vi "Detect LR.vi"(9 "Side Gyro Data":T1={"Time"=0.0, "Gyro Array Data"=[], "Gyro Negation"=[], "Gyro Data"={"Gyro X"=0.0, "Gyro Y"=0.0, "Gyro Z"=0.0}, "Gyro Latency"=0.0, "Normalization Time"=640.0, "Sampling Rate"=0.0}, 10 "Side Event Data":T3={"Event Data"={"LR"={"Phase"="LR", "On"=FALSE, "Last On Time"=0.0, "Duration"=0.0, "Crossing Time"=0.0, "Time since LR"=0.0, "Time Since TSw"=0.0, "Min gyro Z"=0.0, "Time since LR?"=FALSE, "Time since TSw?"=FALSE, "Min gyro Z?"=FALSE, "Crossing?"=FALSE}, "MSt"={"Phase"="MSt", "On"=FALSE, "Last On Time"=0.0, "Duration"=0.0}, "TSt"={"Phase"="TSt", "On"=FALSE, "Last On Time"=0.0, "Duration"=0.0}, "PSw"={"Phase"="PSw", "On"=FALSE, "Last On Time"=0.0, "Duration"=0.0}, "ISw"={"Phase"="ISw", "On"=FALSE, "Last On Time"=0.0, "Duration"=0.0, "Peak Time"=0.0, "Time since LR"=0.0, "Time since ISw"=0.0, "Time since LR?"=FALSE, "Time since ISw?"=FALSE, "Peak?"=FALSE}, "MSw"={"Phase"="MSw", "On"=FALSE, "Last On Time"=0.0, "Duration"=0.0, "Crossing time"=0.0, "Time since LR"=0.0, "Time since MSw"=0.0, "Time since ISw"=0.0, "Time since LR?"=FALSE, "Time since MSw?"=FALSE, "Time since ISw?"=FALSE, "Crossing?"=FALSE}, "TSw"={"Phase"="TSw", "On"=FALSE, "Last On Time"=0.0, "Duration"=0.0, "Peak time"=0.0, "Time since LR"=0.0, "Time since TSw"=0.0, "Time since LR?"=FALSE, "Time since TSw?"=FALSE, "Peak?"=FALSE}}, "Mean Cycle Duration"=0.0, "Event Detected?"=FALSE, "Last Event Detected"=0, "Num Cycles"=0.0, "GPD Log"=refnum, "Last Event Time"=0.0}, 11 "GPD Parameters":T4={"% Cycle Delay"=0.0, "Min % Cycle LR to ISw "=0.0, "Min % Cycle LR to MSw"=0.0, "Min % Cycle LR to TSw"=0.0, "Max % Cycle ISw to MSw"=0.0, "Min % Cycle TSw to LR"=0.0, "Max % Cycle TSw to LR"=0.0, "LR Min Gyro Z Threshold"=0.0, "LR Min Gyro Z Width"=0.0, "ISw Peak Threshold"=0.0, "ISw Peak Width"=0.0, "TSw Valley Threshold"=0.0, "TSw Valley Width (ms)"=7.0, "Max Cycle Time (s)"=0.0, "Mean Computation Window"=0.0, "CP subject?"=FALSE}) -> (1 "Side Gyro Data":T1={"Time"=0.0, "Gyro Array Data"=[], "Gyro Negation"=[], "Gyro Data"={"Gyro X"=0.0, "Gyro Y"=0.0, "Gyro Z"=0.0}, "Gyro Latency"=0.0, "Normalization Time"=640.0, "Sampling Rate"=0.0}, 2 "Side Event Data":T3={"Event Data"={"LR"={"Phase"="LR", "On"=FALSE, "Last On Time"=0.0, "Duration"=0.0, "Crossing Time"=0.0, "Time since LR"=0.0, "Time Since TSw"=0.0, "Min gyro Z"=0.0, "Time since LR?"=FALSE, "Time since TSw?"=FALSE, "Min gyro Z?"=FALSE, "Crossing?"=FALSE}, "MSt"={"Phase"="MSt", "On"=FALSE, "Last On Time"=0.0, "Duration"=0.0}, "TSt"={"Phase"="TSt", "On"=FALSE, "Last On Time"=0.0, "Duration"=0.0}, "PSw"={"Phase"="PSw", "On"=FALSE, "Last On Time"=0.0, "Duration"=0.0}, "ISw"={"Phase"="ISw", "On"=FALSE, "Last On Time"=0.0, "Duration"=0.0, "Peak Time"=0.0, "Time since LR"=0.0, "Time since ISw"=0.0, "Time since LR?"=FALSE, "Time since ISw?"=FALSE, "Peak?"=FALSE}, "MSw"={"Phase"="MSw", "On"=FALSE, "Last On Time"=0.0, "Duration"=0.0, "Crossing time"=0.0, "Time since LR"=0.0, "Time since MSw"=0.0, "Time since ISw"=0.0, "Time since LR?"=FALSE, "Time since MSw?"=FALSE, "Time since ISw?"=FALSE, "Crossing?"=FALSE}, "TSw"={"Phase"="TSw", "On"=FALSE, "Last On Time"=0.0, "Duration"=0.0, "Peak time"=0.0, "Time since LR"=0.0, "Time since TSw"=0.0, "Time since LR?"=FALSE, "Time since TSw?"=FALSE, "Peak?"=FALSE}}, "Mean Cycle Duration"=0.0, "Event Detected?"=FALSE, "Last Event Detected"=0, "Num Cycles"=0.0, "GPD Log"=refnum, "Last Event Time"=0.0}, 3 "GPD Parameters":T4={"% Cycle Delay"=0.0, "Min % Cycle LR to ISw "=0.0, "Min % Cycle LR to MSw"=0.0, "Min % Cycle LR to TSw"=0.0, "Max % Cycle ISw to MSw"=0.0, "Min % Cycle TSw to LR"=0.0, "Max % Cycle TSw to LR"=0.0, "LR Min Gyro Z Threshold"=0.0, "LR Min Gyro Z Width"=0.0, "ISw Peak Threshold"=0.0, "ISw Peak Width"=0.0, "TSw Valley Threshold"=0.0, "TSw Valley Width (ms)"=7.0, "Max Cycle Time (s)"=0.0, "Mean Computation Window"=0.0, "CP subject?"=FALSE}, 4 "LR Detected?":bool)   [LabVIEW 2019]
uses:
  Controls/Gyro Side Data.ctl
  Controls/Gyro Negation.ctl
  Controls/GPD Side Parameters.ctl
  Controls/Side Event Data.ctl
  <vilib>/ptbypt/NI_PtbyPt.lvlib
panel:
  out "LR at about 7 sec":bool
  out "output cluster":T5
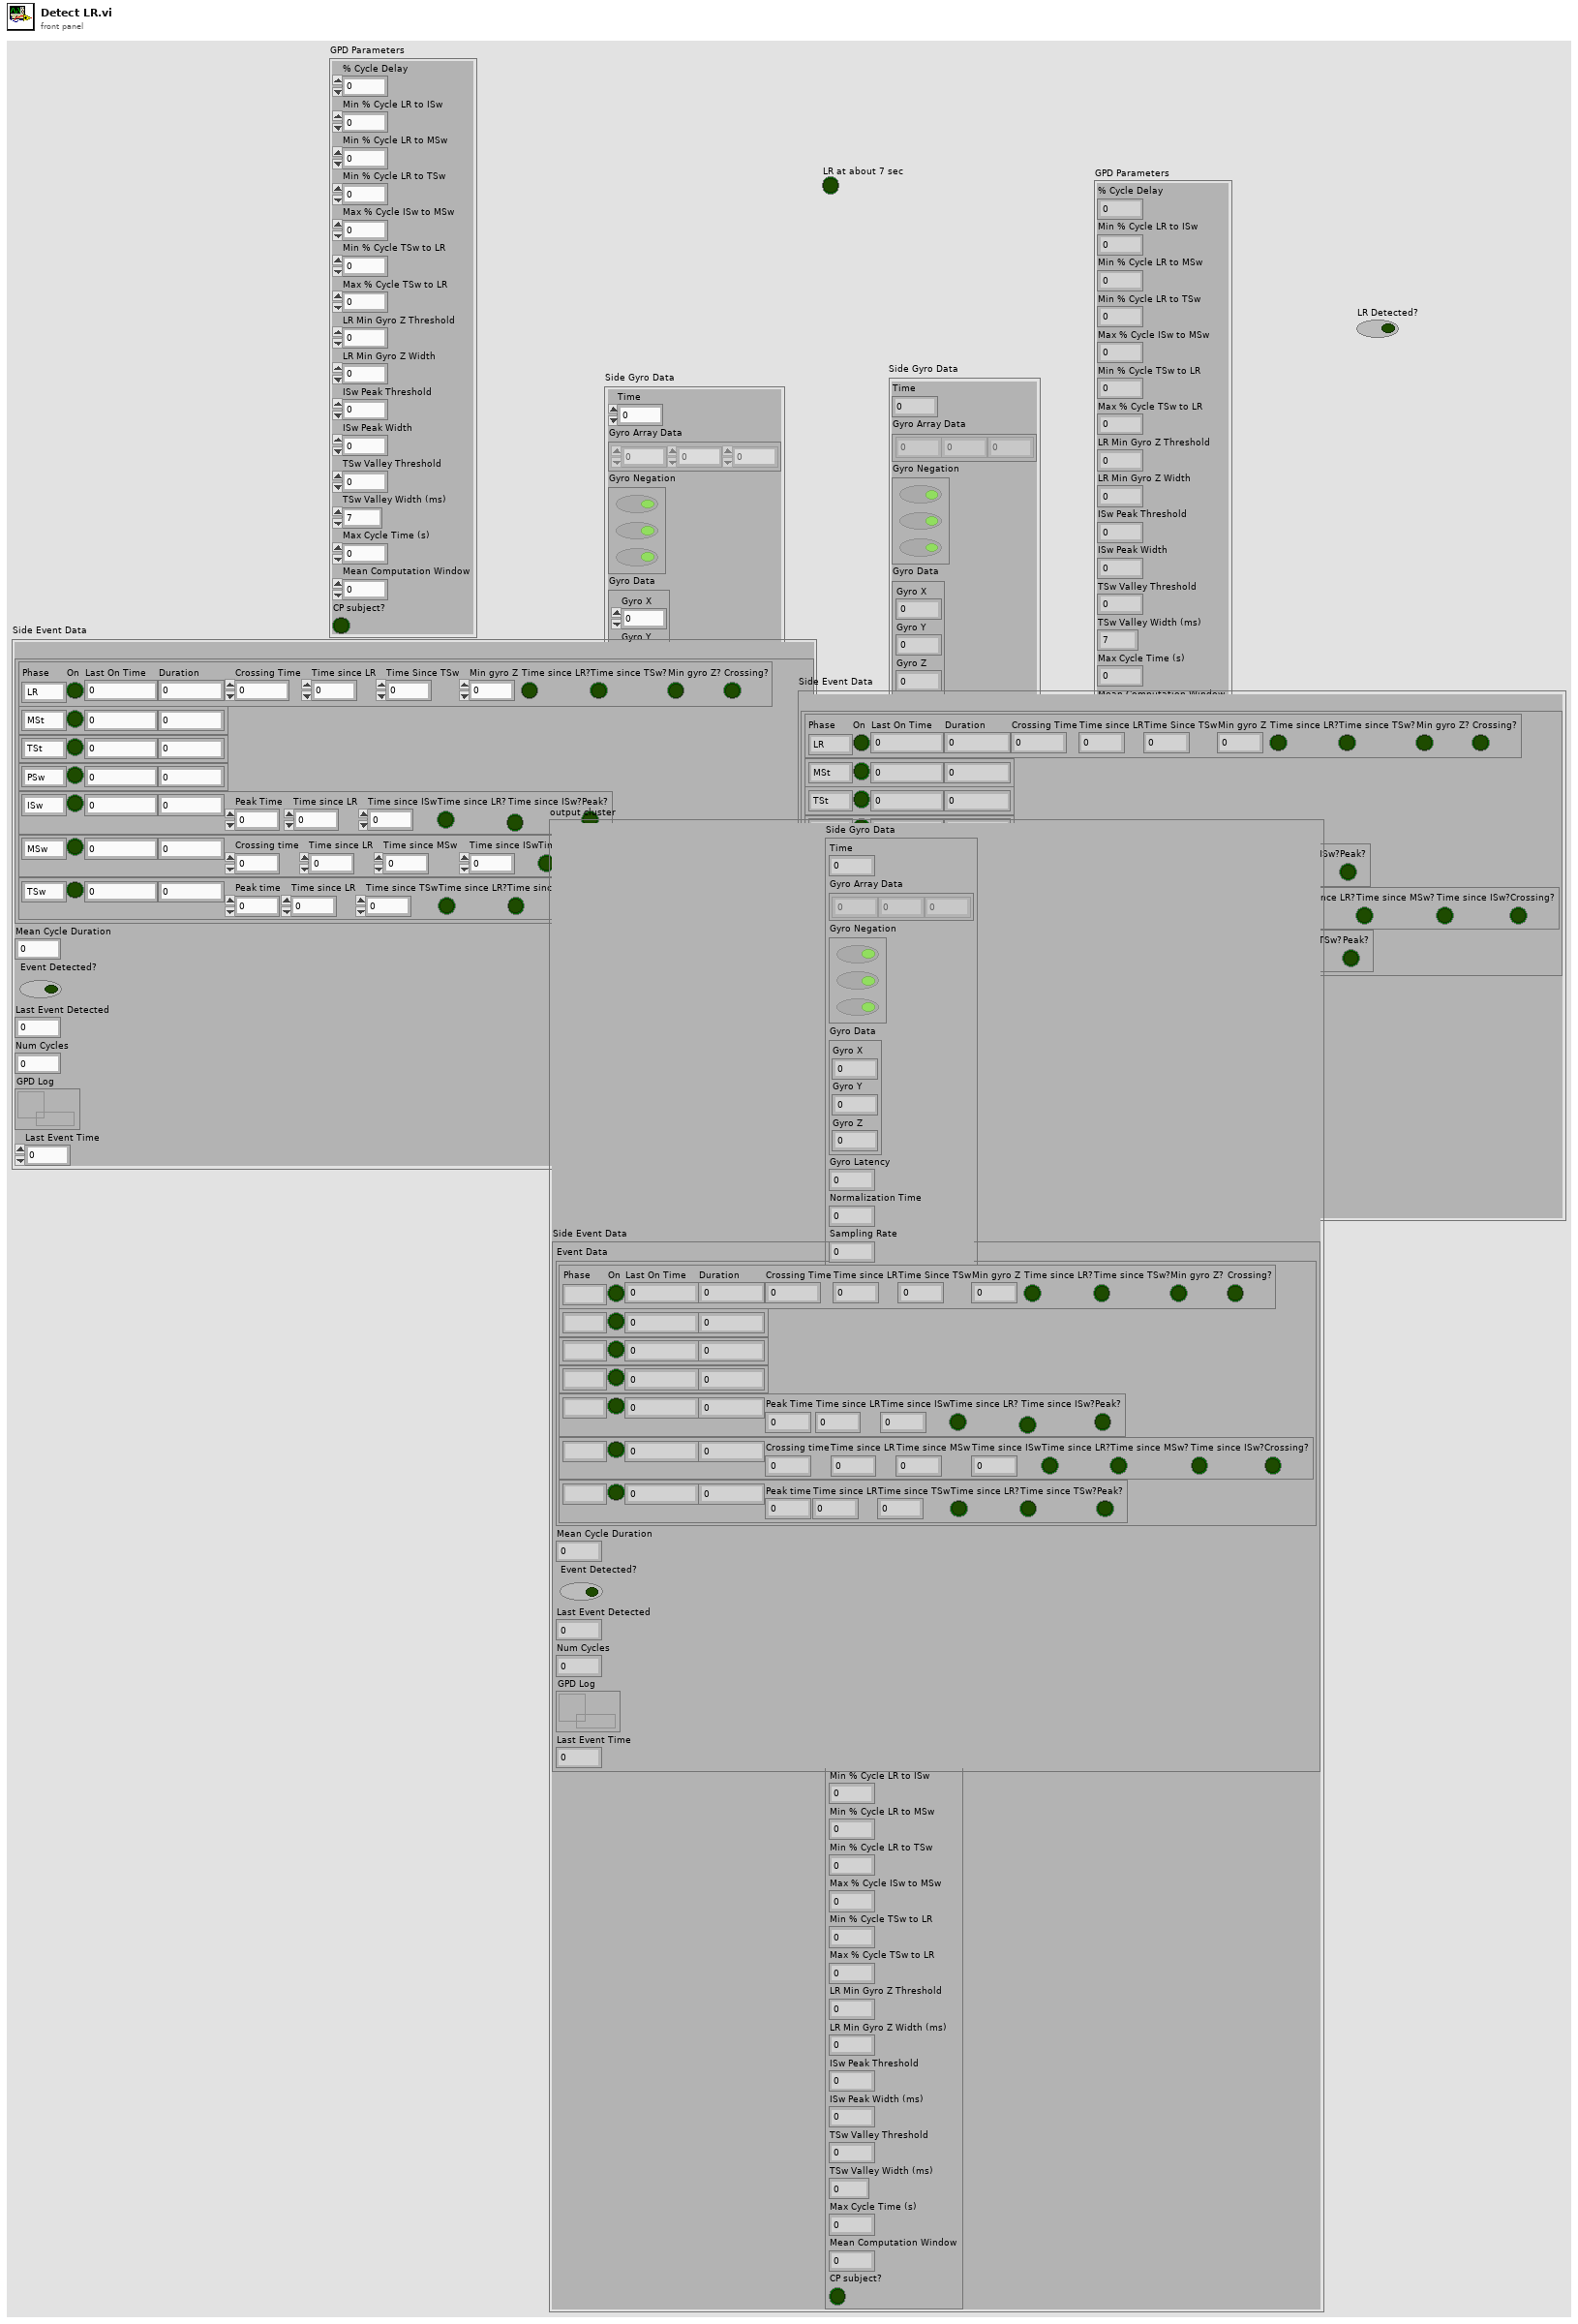
[diagram p1: front panel]
types:
  T1 = typedef "Gyro Side Data.ctl" = cluster{"Time":dbl, "Gyro Array Data":dbl[], "Gyro Negation":T2, "Gyro Data":cluster{"Gyro X":dbl, "Gyro Y":dbl, "Gyro Z":dbl}, "Gyro Latency":dbl, "Normalization Time":dbl, "Sampling Rate":dbl}
  T2 = typedef "Gyro Negation.ctl" = bool[]
  T3 = typedef "Side Event Data.ctl" = cluster{"Event Data":cluster{"LR":cluster{"Phase":string, "On":bool, "Last On Time":dbl, "Duration":dbl, "Crossing Time":dbl, "Time since LR":dbl, "Time Since TSw":dbl, "Min gyro Z":dbl, "Time since LR?":bool, "Time since TSw?":bool, "Min gyro Z?":bool, "Crossing?":bool}, "MSt":cluster{"Phase":string, "On":bool, "Last On Time":dbl, "Duration":dbl}, "TSt":cluster{"Phase":string, "On":bool, "Last On Time":dbl, "Duration":dbl}, "PSw":cluster{"Phase":string, "On":bool, "Last On Time":dbl, "Duration":dbl}, "ISw":cluster{"Phase":string, "On":bool, "Last On Time":dbl, "Duration":dbl, "Peak Time":dbl, "Time since LR":dbl, "Time since ISw":dbl, "Time since LR?":bool, "Time since ISw?":bool, "Peak?":bool}, "MSw":cluster{"Phase":string, "On":bool, "Last On Time":dbl, "Duration":dbl, "Crossing time":dbl, "Time since LR":dbl, "Time since MSw":dbl, "Time since ISw":dbl, "Time since LR?":bool, "Time since MSw?":bool, "Time since ISw?":bool, "Crossing?":bool}, "TSw":cluster{"Phase":string, "On":bool, "Last On Time":dbl, "Duration":dbl, "Peak time":dbl, "Time since LR":dbl, "Time since TSw":dbl, "Time since LR?":bool, "Time since TSw?":bool, "Peak?":bool}}, "Mean Cycle Duration":dbl, "Event Detected?":bool, "Last Event Detected":i32, "Num Cycles":dbl, "GPD Log":refnum<queue>, "Last Event Time":dbl}
  T4 = typedef "GPD Side Parameters.ctl" = cluster{"% Cycle Delay":dbl, "Min % Cycle LR to ISw ":dbl, "Min % Cycle LR to MSw":dbl, "Min % Cycle LR to TSw":dbl, "Max % Cycle ISw to MSw":dbl, "Min % Cycle TSw to LR":dbl, "Max % Cycle TSw to LR":dbl, "LR Min Gyro Z Threshold":dbl, "LR Min Gyro Z Width":dbl, "ISw Peak Threshold":dbl, "ISw Peak Width":dbl, "TSw Valley Threshold":dbl, "TSw Valley Width (ms)":dbl, "Max Cycle Time (s)":dbl, "Mean Computation Window":dbl, "CP subject?":bool}
  T5 = cluster{"Side Gyro Data":T1, "Side Event Data":T3, "GPD Parameters":T4}
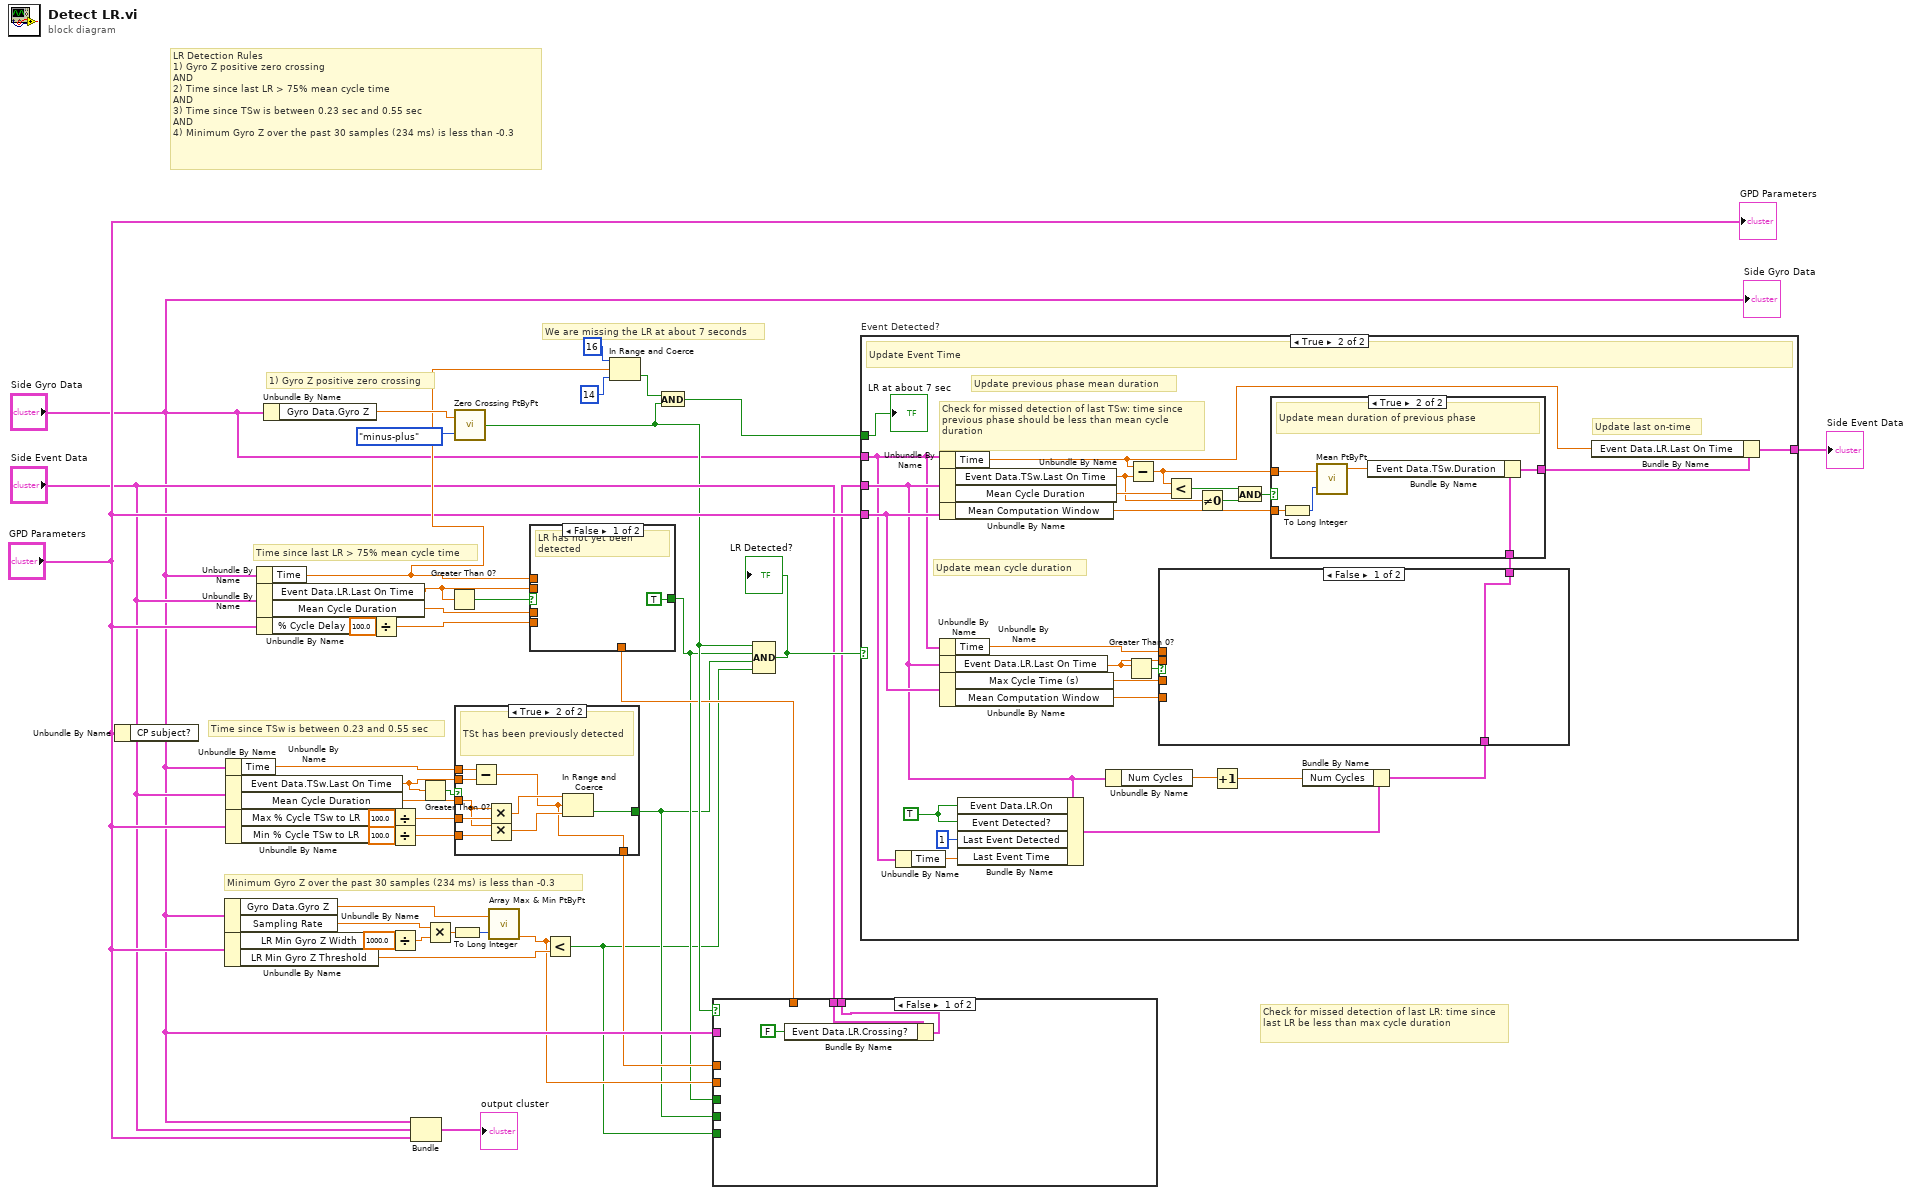
[diagram p0: block diagram]
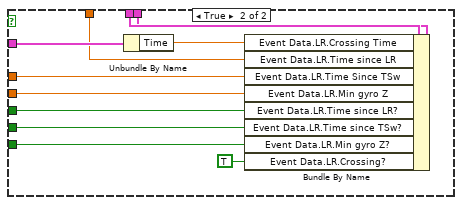
[diagram p2: hidden frame]
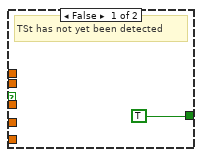
[diagram p3: hidden frame]
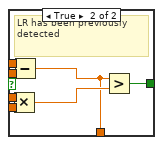
[diagram p4: hidden frame]
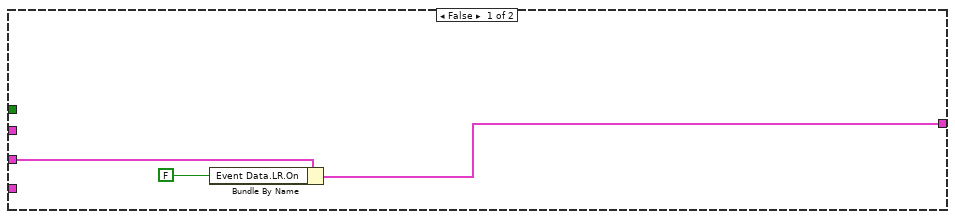
[diagram p5: hidden frame]
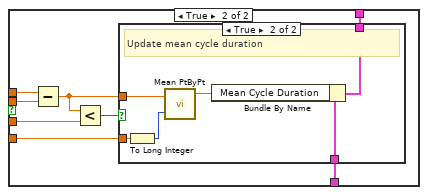
[diagram p6: hidden frame]
diagram:
  # "Check for missed detection of last LR: time since last LR be less than max cycle duration"
  # "Minimum Gyro Z over the past 30 samples (234 ms) is less than -0.3"
  # "Time since TSw is between 0.23 and 0.55 sec"
  # "Time since last LR > 75% mean cycle time"
  # "We are missing the LR at about 7 seconds"
  # "1) Gyro Z positive zero crossing"
  # "LR Detection Rules\n1) Gyro Z positive zero crossing\nAND\n2) Time since last LR > 75% mean cycle time\nAND\n3) Time since TSw is between 0.23 sec and 0.55 sec\nAND\n4) Minimum Gyro Z over the past 30 samples (234 ms) is less than -0.3"
  n1 = Unbundle By Name("GPD Parameters") -> ()  [unwired: 1 out]
  n2 = Unbundle By Name("Side Gyro Data") -> ("Gyro Data.Gyro Z"=w20:dbl, "Sampling Rate"=w16:dbl)
  n3 = Unbundle By Name("GPD Parameters") -> ("LR Min Gyro Z Width"=w18:dbl, "LR Min Gyro Z Threshold"=w13:dbl)
  n4 = Unbundle By Name("Side Gyro Data") -> ("Time"=w28:dbl)
  n5 = Unbundle By Name("Side Event Data") -> ("Event Data.TSw.Last On Time"=w11:dbl, "Mean Cycle Duration"=w22:dbl)
  n6 = Unbundle By Name("GPD Parameters") -> ("Max % Cycle TSw to LR"=w25:dbl, "Min % Cycle TSw to LR"=w24:dbl)
  n7 = Unbundle By Name("Side Gyro Data") -> ("Time"=w31:dbl)
  n8 = Unbundle By Name("Side Event Data") -> ("Event Data.LR.Last On Time"=w37:dbl, "Mean Cycle Duration"=w34:dbl)
  n9 = Unbundle By Name("GPD Parameters") -> ("% Cycle Delay"=w33:dbl)
  n10 = Unbundle By Name("Side Gyro Data") -> ("Gyro Data.Gyro Z"=w43:dbl)
  n11 = Divide(x=w33, y=100.0) -> (x/y=w35:dbl)
  n12 = Divide(x=w25, y=100.0) -> (x/y=w23:dbl)
  n13 = Divide(x=w24, y=100.0) -> (x/y=w21:dbl)
  n14 = Divide(x=w18, y=1000.0) -> (x/y=w17:dbl)
  n15 = Bundle("Side Gyro Data"="Side Gyro Data", "Side Event Data"="Side Event Data", "GPD Parameters"="GPD Parameters") -> (→"output cluster":T5)  [unwired: 1 in]
  n16 = Greater Than 0?(x=w11) -> (x > 0?=w12:bool)
  n17 = Multiply(x=w16, y=w17) -> (x*y=w15:dbl)
  n18 = Greater Than 0?(x=w37) -> (x > 0?=w36:bool)
  n19 = To Long Integer(number=w15) -> (32bit integer=w14:i32)
  n20 = call <vilib>:"Zero Crossing PtByPt.vi"("direction"=enum16{"either", "minus-plus", "plus-minus"}."minus-plus", "input data point"=w43) -> ("crossing"=w8:bool)  [unwired: 1 in]
  n21 = case shown="True" w12 {
    tunnel: w28 -> [_ w55]
    tunnel: w11 -> [_ w54]
    tunnel: w23 -> [_ w53]
    tunnel: w22 -> [_ w52]
    tunnel: w21 -> [_ w51]
    tunnel: [TRUE w48] -> w2
    tunnel: [_ w47] -> w5
    frame False {
      # "TSt has not yet been detected"
    }
    frame True {
      # "TSt has been previously detected"
      n22 = Subtract(x=w55, y=w54) -> (x-y=w47:dbl)
      n23 = Multiply(x=w52, y=w53) -> (x*y=w50:dbl)
      n24 = Multiply(x=w52, y=w51) -> (x*y=w49:dbl)
      n25 = In Range and Coerce(upper limit=w50, x=w47, lower limit=w49) -> (In Range?=w48:bool)  [unwired: 1 out]
    }
  }
  n26 = call <vilib>:"Array Max & Min PtByPt.vi"("input data point"=w20, "sample length"=w14) -> ("min value"=w4:dbl)  [unwired: 1 in, 4 out]
  n27 = case shown="False" w36 {
    tunnel: w34 -> [_ w63]
    tunnel: w35 -> [_ w62]
    tunnel: w31 -> [_ w61]
    tunnel: w37 -> [_ w60]
    tunnel: [TRUE w59] -> w3
    tunnel: [_ w57] -> w6
    frame False {
      # "LR has not yet been detected"
    }
    frame True {
      # "LR has been previously detected"
      n28 = Multiply(x=w63, y=w62) -> (x*y=w58:dbl)
      n29 = Subtract(x=w61, y=w60) -> (x-y=w57:dbl)
      n30 = Greater?(x=w57, y=w58) -> (0:w59:bool)
    }
  }
  n31 = Less?(x=w4, y=w13) -> (x < y?=w1:bool)
  n32 = In Range and Coerce(upper limit=16, x=w31, lower limit=14) -> (In Range?=w39:bool)  [unwired: 1 out]
  n33 = And(x=w39, y=w8) -> (x .and. y?=w38:bool)
  n34 = case shown="False" w8 {
    tunnel: "Side Event Data" -> [w65 w77]
    tunnel: [w64 w76] -> w9
    tunnel: "Side Gyro Data" -> [_ w75]
    tunnel: w6 -> [_ w73]
    tunnel: w5 -> [_ w72]
    tunnel: w4 -> [_ w71]
    tunnel: w3 -> [_ w70]
    tunnel: w2 -> [_ w69]
    tunnel: w1 -> [_ w68]
    frame False {
      n35 = Bundle By Name(cluster=w65, "Event Data.LR.Crossing?"=FALSE) -> (w64:T3)
    }
    frame True {
      n36 = Unbundle By Name(w75) -> ("Time"=w74:dbl)
      n37 = Bundle By Name(cluster=w77, "Event Data.LR.Crossing Time"=w74, "Event Data.LR.Time since LR"=w73, "Event Data.LR.Time Since TSw"=w72, "Event Data.LR.Min gyro Z"=w71, "Event Data.LR.Time since LR?"=w70, "Event Data.LR.Time since TSw?"=w69, "Event Data.LR.Min gyro Z?"=w68, "Event Data.LR.Crossing?"=TRUE) -> (w76:T3)
    }
  }
  n38 = Compound Arithmetic op=AND(w8, w3, w2, w1) -> (w30:bool)
  "LR Detected?" <- w30
  n39 = case "Event Detected?" shown="True" w30 {
    tunnel: w9 -> [w80 w92]
    tunnel: [w79 w96] -> w45
    tunnel: "Side Gyro Data" -> [_ w84]
    tunnel: "GPD Parameters" -> [_ w100]
    tunnel: w38 -> [_ w83]
    frame False {
      n40 = Bundle By Name(cluster=w80, "Event Data.LR.On"=FALSE) -> (w79:T3)
    }
    frame True {
      w106 = TRUE
      # "Update last on-time"
      # "Check for missed detection of last TSw: time since previous phase should be less than mean cycle duration"
      # "Update mean cycle duration"
      # "Update previous phase mean duration"
      # "Update Event Time"
      n41 = Unbundle By Name(w84) -> ("Time"=w85:dbl)
      n42 = Unbundle By Name(w84) -> ("Time"=w104:dbl)
      n43 = Unbundle By Name(w92) -> ("Event Data.TSw.Last On Time"=w86:dbl, "Mean Cycle Duration"=w90:dbl)
      n44 = Unbundle By Name(w100) -> ("Mean Computation Window"=w94:dbl)
      n45 = Unbundle By Name(w84) -> ("Time"=w101:dbl)
      n46 = Unbundle By Name(w92) -> ("Event Data.LR.Last On Time"=w81:dbl)
      n47 = Unbundle By Name(w100) -> ("Max Cycle Time (s)"=w99:dbl, "Mean Computation Window"=w93:dbl)
      n48 = Bundle By Name(cluster=w92, "Event Data.LR.On"=w106, "Event Detected?"=w106, "Last Event Detected"=1, "Last Event Time"=w85) -> (w103:T3)
      n49 = Unbundle By Name(w92) -> ("Num Cycles"=w91:dbl)
      n50 = Greater Than 0?(x=w81) -> (x > 0?=w82:bool)
      n51 = Subtract(x=w104, y=w86) -> (x-y=w107:dbl)
      n52 = Less?(x=w107, y=w90) -> (x < y?=w88:bool)
      n53 = Not Equal To 0?(x=w86) -> (x != 0?=w89:bool)
      n54 = Increment(x=w91) -> (x+1=w102:dbl)
      n55 = And(x=w88, y=w89) -> (x .and. y?=w87:bool)
      n56 = Bundle By Name(cluster=w103, "Num Cycles"=w102) -> (w98:T3)
      n57 = case shown="False" w82 {
        tunnel: w101 -> [_ w116]
        tunnel: w81 -> [_ w115]
        tunnel: w99 -> [_ w114]
        tunnel: w98 -> [w108 w111]
        tunnel: [w108 w110] -> w97
        tunnel: w93 -> [_ w109]
        frame False {
        }
        frame True {
          n58 = Subtract(x=w116, y=w115) -> (x-y=w112:dbl)
          n59 = Less?(x=w112, y=w114) -> (x < y?=w113:bool)
          n60 = case shown="True" w113 {
            tunnel: w112 -> [_ w123]
            tunnel: w111 -> [w117 w122]
            tunnel: [w117 w120] -> w110
            tunnel: w109 -> [_ w119]
            frame False {
            }
            frame True {
              # "Update mean cycle duration"
              n61 = To Long Integer(number=w119) -> (32bit integer=w118:i32)
              n62 = call <vilib>:"Mean PtByPt.vi"("x"=w123, "sample length"=w118) -> ("mean"=w121:dbl)  [unwired: 2 in, 1 out]
              n63 = Bundle By Name(cluster=w122, "Mean Cycle Duration"=w121) -> (w120:T3)
            }
          }
        }
      }
      n64 = case shown="True" w87 {
        tunnel: w107 -> [_ w130]
        tunnel: w97 -> [w124 w129]
        tunnel: [w124 w127] -> w95
        tunnel: w94 -> [_ w126]
        frame False {
        }
        frame True {
          # "Update mean duration of previous phase"
          n65 = To Long Integer(number=w126) -> (32bit integer=w125:i32)
          n66 = call <vilib>:"Mean PtByPt.vi"("x"=w130, "sample length"=w125) -> ("mean"=w128:dbl)  [unwired: 2 in, 1 out]
          n67 = Bundle By Name(cluster=w129, "Event Data.TSw.Duration"=w128) -> (w127:T3)
        }
      }
      n68 = Bundle By Name(cluster=w95, "Event Data.LR.Last On Time"=w104) -> (w96:T3)
      "LR at about 7 sec" <- w83
    }
  }
  "Side Event Data" <- w45
  "Side Gyro Data" <- "Side Gyro Data"
  "GPD Parameters" <- "GPD Parameters"
